vi "Camera-Roll.vi"() -> ()   [LabVIEW 2019]
uses:
  <vilib>/Rock Robotics/WPI/Utilities/WPI_GetSetVariantRefNum.vi
  <vilib>/Rock Robotics/SystemInterfaces/DIO/FPGA_DIOPWMChannel.ctl
panel:
  in  "Boolean":bool
  in  "Angle":i32
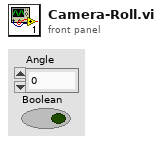
[diagram p1: front panel]
types:
  T1 = typedef "FPGA_DIOPWMChannel.ctl" = enum8{"PWM 0", "PWM 1", "PWM 2", "PWM 3", "PWM 4", "PWM 5", "PWM 6", "PWM 7", "PWM 8", "PWM 9", "PWM MXP 0", "PWM MXP 1", "PWM MXP 2", "PWM MXP 3", "PWM MXP 4", "PWM MXP 5", "PWM MXP 6", "PWM MXP 7", "PWM MXP 8", "PWM MXP 9", "Invalid"}
  T2 = typedef "WPI_ServoDeviceRef.ctl" = cluster{"DeviceStatus":errorcluster, "PWM Channel":T1, "DeadBand":T3}
  T3 = typedef "WPI_PWMDeadband.ctl" = cluster{"Name":string, "maxPositivePwm":i32, "minPositivePwm":i32, "centerPwm":i32, "maxNegativePwm":i32, "minNegativePwm":i32, "angularRange":u16}
  T4 = typedef "WPI_JoystickDevRef.ctl" = cluster{"Device":T5}
  T5 = typedef "WPI_JoystickDeviceEnum.ctl" = enum16{"USB 0", "USB 1", "USB 2", "USB 3", "USB 4", "USB 5"}
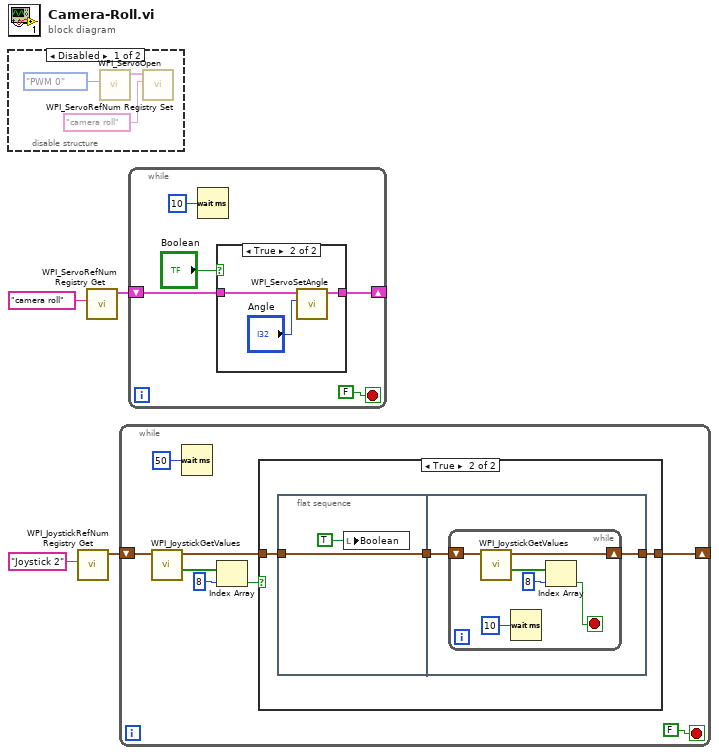
[diagram p0: block diagram]
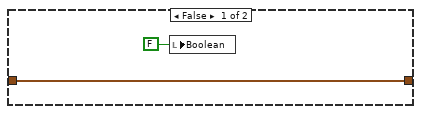
[diagram p2: hidden frame]
diagram:
  n1 = disable-structure shown="Disabled" {
    frame Disabled {
      n2 = call <vilib>:"WPI_ServoOpen.vi"("PWM Channel"=FPGA_DIOPWMChannel."PWM 0") -> ("ServoDeviceRef"=w7:T2)  [unwired: 9 in, 1 out]
      n3 = call <vilib>:"WPI_ServoRefNum Registry Set.vi"("refnum name"="camera roll", "ServoDeviceRef"=w7) -> ()  [unwired: 8 in, 2 out]
    }
    frame Enabled {
    }
  }
  n4 = call <vilib>:"WPI_JoystickRefNum Registry Get.vi"("refnum name"="Joystick 2") -> ("JoystickDevRef"=w1:T4)  [unwired: 9 in, 1 out]
  n5 = call <vilib>:"WPI_ServoRefNum Registry Get.vi"("refnum name"="camera roll") -> ("ServoDeviceRef"=w3:T2)  [unwired: 9 in, 1 out]
  n6 = while {
    shift-right: [w8] -> _
    shift-left: w1 -> [w15]
    stop <- FALSE stop-if-true
    n7 = call <vilib>:"WPI_JoystickGetValues.vi"("JoystickDevRef"=w15) -> ("Buttons"=w14:bool[], "JoystickDevRef"=w10:T4)  [unwired: 6 in, 3 out]
    n8 = Wait (ms)(milliseconds to wait=u32 50) -> ()  [unwired: 1 out]
    n9 = Index Array(array=w14, index=8) -> (element=w12:bool)
    n10 = case shown="True" w12 {
      tunnel: w10 -> [w16 w19]
      tunnel: [w16 w18] -> w8
      frame False {
        n11 = local write "Boolean"(FALSE ("Boolean")) -> ()
      }
      frame True {
        n12 = flat-sequence {
          tunnel: [w21] -> w20
          tunnel: w19 -> [w21]
          tunnel: w20 -> [w24]
          tunnel: [w23] -> w18
          frame #0 {
            n13 = local write "Boolean"(TRUE ("Boolean")) -> ()
          }
          frame #1 {
            n14 = while {
              shift-right: [w29] -> w23
              shift-left: w24 -> [w30]
              stop <- w26 stop-if-true
              n15 = call <vilib>:"WPI_JoystickGetValues.vi"("JoystickDevRef"=w30) -> ("Buttons"=w28:bool[], "JoystickDevRef"=w29:T4)  [unwired: 6 in, 3 out]
              n16 = Wait (ms)(milliseconds to wait=u32 10) -> ()  [unwired: 1 out]
              n17 = Index Array(array=w28, index=8) -> (element=w26:bool)
            }
          }
        }
      }
    }
  }
  n18 = while {
    shift-right: [w32] -> _
    shift-left: w3 -> [w33]
    stop <- FALSE stop-if-true
    n19 = Wait (ms)(milliseconds to wait=u32 10) -> ()  [unwired: 1 out]
    n20 = case shown="True" "Boolean" {
      tunnel: w33 -> [w36 w39]
      tunnel: [w36 w38] -> w32
      frame False {
      }
      frame True {
        n21 = call <vilib>:"WPI_ServoSetAngle.vi"("Angle"="Angle", "ServoDeviceRef"=w39) -> ("ServoDeviceRef"=w38:T2)  [unwired: 8 in, 1 out]
      }
    }
  }
